vi "ManipuLEAPIt.vi"() -> ()   [LabVIEW 2011]
uses:
  <vilib>/LabVIEW Hacker/Leap/Public/Instance VIs/Read 1 Hand Position Velocity.vi
  <vilib>/LabVIEW Hacker/Leap/Public/Gestures/Circle/Instance VIs/Read 1 Circle Progress.vi
  <vilib>/LabVIEW Hacker/Leap/Public/Gestures/Swipe/Instance VIs/Read 1 Swipe Direction.vi
  <vilib>/LabVIEW Hacker/Leap/Public/Gestures/Key Tap/Instance VIs/Read 1 Key Tap Position.vi
  <vilib>/picture/3D Picture Control/NI_3D Picture Control.lvlib
  <vilib>/LabVIEW Hacker/Leap/LVH-Leap.lvlib
panel:
  in  "Start":bool
  in  "stop":bool
  out "Force Field":refnum<vi>(3d-picture)
  # "1 - Press the Play Button\n      (Must be yellow to start)\n2 - Run the VI\n3 - Put your right hand over the LEAP Motion\n4 - Commands:\n    4.1  Move Up: swipe up\n    4.2  Move Down: swipe down\n    4.3  Move Left: swipe left\n    4.4  Move Right: swipe right\n    4.5  Move In:  swipe in\n    4.6  Mve Out:  swipe out\n    4.7  Rezise:  Just move your hand\n    4.8  Rotate left:  do circles\n    4.9  Reset position: tap (any)\n5 - Press stop to move out the application"
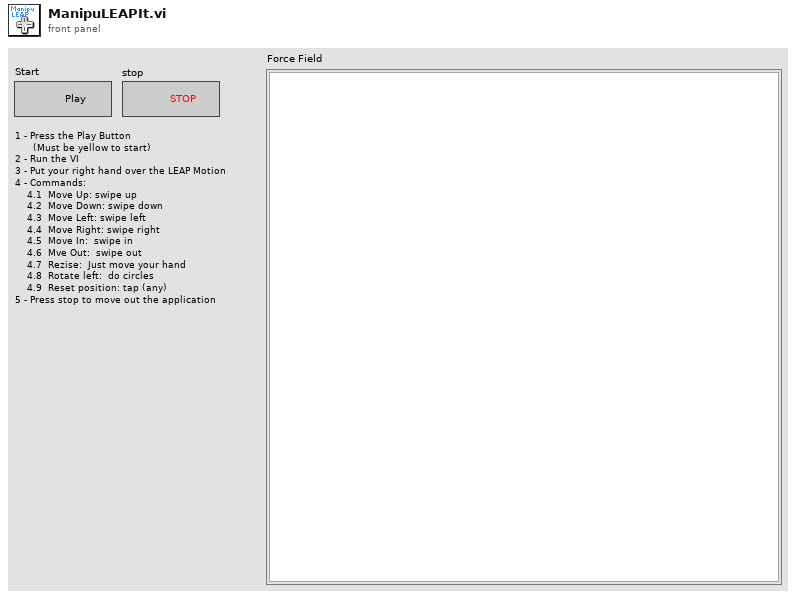
[diagram p1: front panel]
types:
  T1 = typedef "LVH-Leap.lvlib/Leap Handle.ctl" = cluster{"LeapCSharp":refnum<k24>}
  T2 = typedef "LVH-Leap.lvlib/Gesture State.ctl" = enum16{"Invalid", "Start", "Update", "Stop"}
  T3 = typedef "LVH-Leap.lvlib/Swipe Direction.ctl" = enum16{"Left", "Right", "Up", "Down", "In", "Out"}
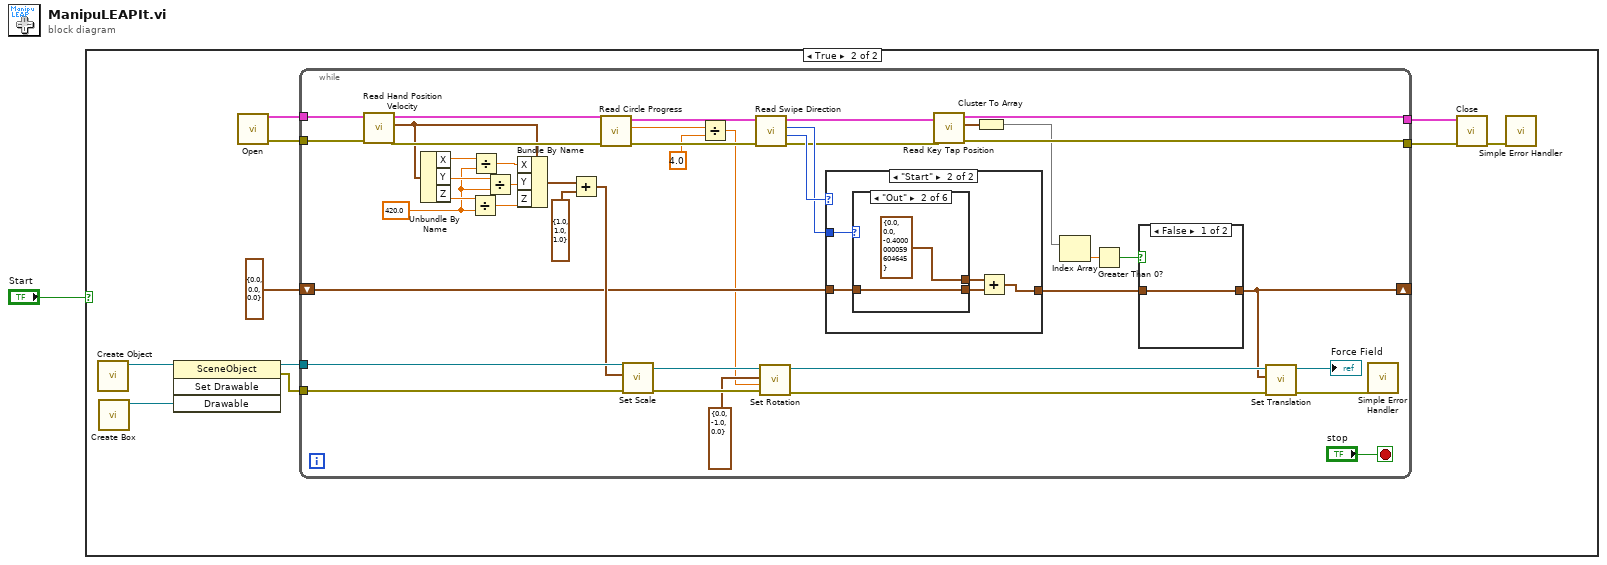
[diagram p0: block diagram]
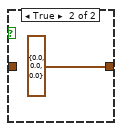
[diagram p3: hidden frame]
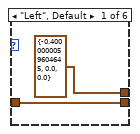
[diagram p5: hidden frame]
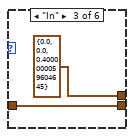
[diagram p6: hidden frame]
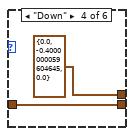
[diagram p7: hidden frame]
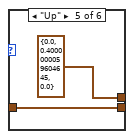
[diagram p8: hidden frame]
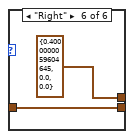
[diagram p9: hidden frame]
diagram:
  n1 = case shown="True" "Start" {
    frame False {
    }
    frame True {
      n2 = call <vilib>:"Create Object.vi"() -> ("Scene:New Object"=w11:refnum<vi>)  [unwired: 10 in, 1 out]
      n3 = call <vilib>:"Create Box.vi"() -> ("New Box Refnum"=w10:refnum<vi>)  [unwired: 10 in, 1 out]
      n4 = invoke class="SceneObject" method="Set Drawable"(reference=w11, "Drawable"=w10) -> (reference out=w9:refnum<vi>, error out=w4:errorcluster)  [unwired: 2 in, 2 out]
      n5 = call <vilib>:"Open.vi"() -> ("Error Out"=w7:errorcluster, "Leap Handle"=w8:T1)  [unwired: 10 in]
      n6 = while {
        tunnel: w9 -> [w33]
        tunnel: w8 -> [w49]
        tunnel: w7 -> [w48]
        tunnel: [w18] -> w6
        tunnel: [w19] -> w5
        tunnel: w4 -> [w32]
        shift-right: [w12] -> _
        shift-left: cluster{"X":sgl, "Y":sgl, "Z":sgl} {"X"=0.0, "Y"=0.0, "Z"=0.0} ("Axis") -> [w25]
        stop <- "stop" stop-if-true
        w39 = 420.0 ("y")
        n7 = call-poly <vilib>:"Read Hand Position Velocity.vi"("Error In"=w48, "Leap Handle"=w49) -> ("Error Out"=w41:errorcluster, "Hand Position"=w36:cluster{"X":sgl, "Y":sgl, "Z":sgl}, "Leap Handle"=w42:T1)  [unwired: 6 in, 1 out]
        n8 = Unbundle By Name(w36) -> ("X"=w47:sgl, "Y"=w46:sgl, "Z"=w45:sgl)
        n9 = Divide(x=w45, y=w39) -> (x/y=w43:dbl)
        n10 = Divide(x=w47, y=w39) -> (x/y=w44:dbl)
        n11 = Divide(x=w46, y=w39) -> (x/y=w40:dbl)
        n12 = Bundle By Name(cluster=w36, "X"=w44, "Y"=w40, "Z"=w43) -> (w38:cluster{"X":sgl, "Y":sgl, "Z":sgl})
        n13 = Add(x=w38, y=cluster{"X":sgl, "Y":sgl, "Z":sgl} {"X"=1.0, "Y"=1.0, "Z"=1.0} ("Scale")) -> (x+y=w30:cluster{"X":sgl, "Y":sgl, "Z":sgl})
        n14 = call-poly <vilib>:"Read Circle Progress.vi"("Error In"=w41, "Leap Handle"=w42) -> ("Error Out"=w28:errorcluster, "Circle Progress"=w23:dbl, "Leap Handle"=w29:T1)  [unwired: 6 in, 1 out]
        n15 = call <vilib>:"Set Scale.vi"("error in (no error)"=w32, "Scale"=w30, "Scene Object"=w33) -> ("error out"=w52:errorcluster, "Scaled Object"=w53:refnum<vi>)  [unwired: 7 in]
        n16 = Divide(x=w23, y=4.0) -> (x/y=w24:dbl)
        n17 = call-poly <vilib>:"Read Swipe Direction.vi"("Error In"=w28, "Leap Handle"=w29) -> ("Error Out"=w20:errorcluster, "Gesture State"=w27:T2, "Swipe Direction"=w26:T3, "Leap Handle"=w21:T1)  [unwired: 6 in]
        n18 = call <vilib>:"Set Rotation.vi"("error in (no error)"=w52, "Angle"=w24, "Axis"=cluster{"X":sgl, "Y":sgl, "Z":sgl} {"X"=0.0, "Y"=-1.0, "Z"=0.0}, "Scene Object"=w53) -> ("error out"=w50:errorcluster, "Rotated Scene Object"=w51:refnum<vi>)  [unwired: 6 in]
        n19 = case shown="\"Start\"" w27 {
          tunnel: w26 -> [_ w62]
          tunnel: w25 -> [w57 w61]
          tunnel: [w57 w58] -> w13
          frame "Invalid", Default {
          }
          frame "Start" {
            n20 = case shown="\"Out\"" w62 {
              tunnel: w61 -> [w64 w66 w67 w70 w71 w74]
              tunnel: [w64 w66 w67 w70 w71 w74] -> w60
              tunnel: [cluster{"X":sgl, "Y":sgl, "Z":sgl} {"X"=-0.4, "Y"=0.0, "Z"=0.0} ("y") cluster{"X":sgl, "Y":sgl, "Z":sgl} {"X"=0.0, "Y"=0.0, "Z"=-0.4} ("y") cluster{"X":sgl, "Y":sgl, "Z":sgl} {"X"=0.0, "Y"=0.0, "Z"=0.4} ("y") cluster{"X":sgl, "Y":sgl, "Z":sgl} {"X"=0.0, "Y"=-0.4, "Z"=0.0} ("y") cluster{"X":sgl, "Y":sgl, "Z":sgl} {"X"=0.0, "Y"=0.4, "Z"=0.0} ("y") cluster{"X":sgl, "Y":sgl, "Z":sgl} {"X"=0.4, "Y"=0.0, "Z"=0.0} ("y")] -> w59
              frame "Left", Default {
              }
              frame "Out" {
              }
              frame "In" {
              }
              frame "Down" {
              }
              frame "Up" {
              }
              frame "Right" {
              }
            }
            n21 = Add(x=w59, y=w60) -> (x+y=w58:cluster{"X":sgl, "Y":sgl, "Z":sgl})
          }
        }
        n22 = call-poly <vilib>:"Read Key Tap Position.vi"("Error In"=w20, "Leap Handle"=w21) -> ("Error Out"=w19:errorcluster, "Key Tap Position"=w17:cluster{"X":sgl, "Y":sgl, "Z":sgl}, "Leap Handle"=w18:T1)  [unwired: 6 in, 1 out]
        n23 = Cluster To Array(cluster=w17) -> (array=w16:sgl[])
        n24 = Index Array(array=w16) -> (element=w15:sgl)  [unwired: 1 in]
        n25 = Greater Than 0?(x=w15) -> (x > 0?=w14:bool)
        n26 = case shown="False" w14 {
          tunnel: w13 -> [w55 _]
          tunnel: [w55 cluster{"X":sgl, "Y":sgl, "Z":sgl} {"X"=0.0, "Y"=0.0, "Z"=0.0} ("Axis")] -> w12
          frame False {
          }
          frame True {
          }
        }
        n27 = call <vilib>:"Set Translation.vi"("error in (no error)"=w50, "Translation"=w12, "Scene Object"=w51) -> ("error out"=w31:errorcluster, "Translated Object"=→"Force Field":refnum<vi>)  [unwired: 7 in]
        n28 = call <vilib>:"Simple Error Handler.vi"("error in (no error)"=w31) -> ()  [unwired: 4 in, 5 out]
      }
      n29 = call <vilib>:"Close.vi"("Error In"=w5, "Leap Handle"=w6) -> ("Error Out"=w3:errorcluster)  [unwired: 9 in]
      n30 = call <vilib>:"Simple Error Handler.vi"("error in (no error)"=w3) -> ()  [unwired: 4 in, 5 out]
    }
  }
